vi "HandleClients.vi"(8 "error in (no error)":errorcluster, 11 "GuiderSetup in":refnum<class "GuiderSetup.lvclass">) -> (0 "error out":errorcluster, 3 "GuiderSetup out":refnum<class "GuiderSetup.lvclass">)   [LabVIEW 2018, in "GuiderSetup.lvclass"]
uses:
  GuiderSetup.lvclass
  C:/Users/devstaff/sparc4/s4gui/Versao ZeroMQ REQ-REP/SPARC4_GUI -v1.0.8 - reconhecimento do ACK do ACS/S4GUI/S4GUI.lvclass
  GuiderSetup.lvclass/GuiderSetup.ctl
  S4GUI/S4GUI.lvclass/S4GUI.ctl
  Instrument/Instrument.lvclass/Instrument.ctl
  Device/Optics/Optics.lvclass/Optics.ctl
  Device/Optics/Opt_Continuous/Opt_Continuous.lvclass
  C:/Users/devstaff/sparc4/s4gui/Versao ZeroMQ REQ-REP/SPARC4_GUI -v1.0.8 - reconhecimento do ACK do ACS/Device/Optics/Optics.lvclass
  Instrument/Instrument.lvclass
  Client_s4gui/Client_s4gui.lvclass
  PublisherGS/PublisherGS.lvclass
  AG/AG.lvclass
  S4GUI/S4GUI.lvclass
  Device/Optics/Optics.lvclass
  StateMachine/State Machine.lvclass
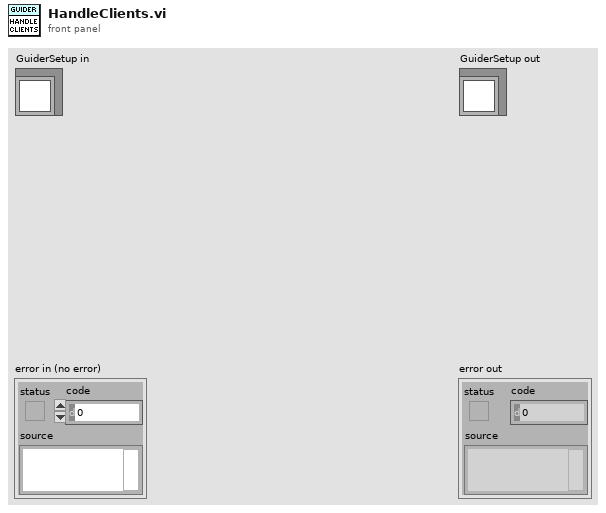
[diagram p1: front panel]
types:
  T1 = cluster{"FocusPhot":dbl, "FocusPolar":dbl, "FocusEffic":dbl, "FocusInstrum":dbl, "ICS":bool, "AG":bool, "broker":string, "timestamp":string, "FocusPos":dbl, "MirrorPos":dbl}
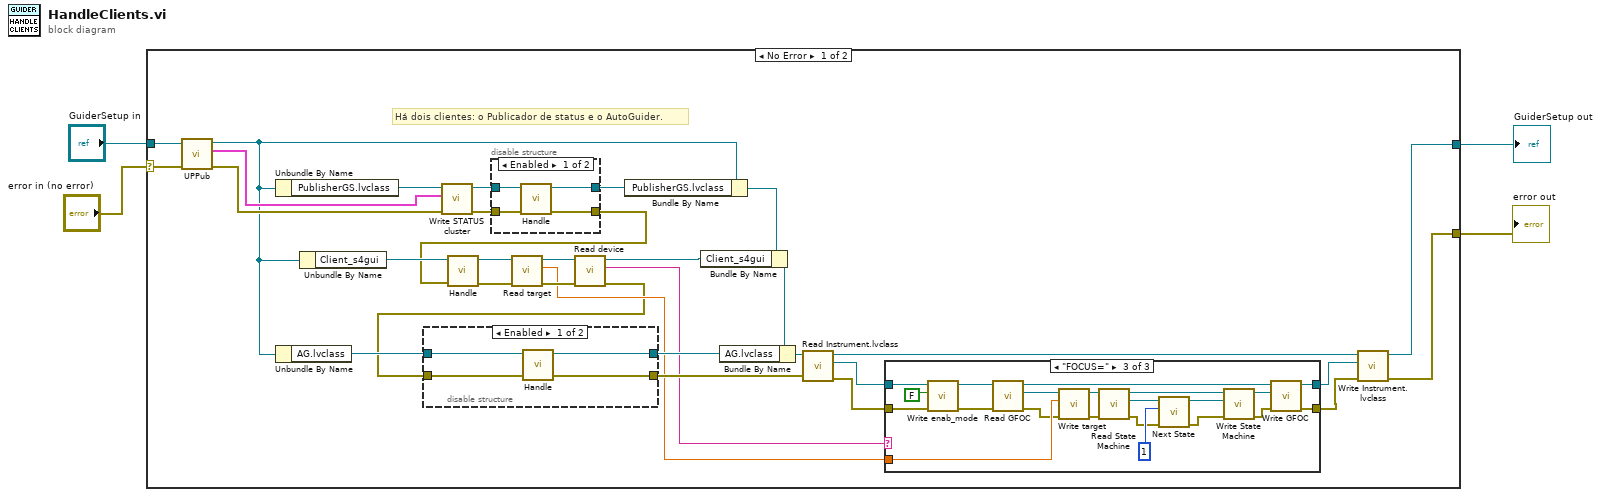
[diagram p0: block diagram]
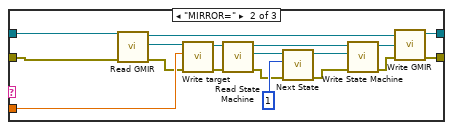
[diagram p3: hidden frame]
diagram:
  n1 = case shown="No Error" "error in (no error)" {
    selector: "error in (no error)" -> [w35 w90]
    tunnel: "GuiderSetup in" -> [w36 w91]
    tunnel: [w20 w91] -> w2
    tunnel: [w18 w90] -> w1
    frame No Error {
      # "Há dois clientes: o Publicador de status e o AutoGuider."
      n2 = call-dynamic "UPPub.vi"("error in (no error)"=w35, "GuiderSetup in"=w36) -> ("error out"=w31:errorcluster, "STATUS cluster"=w32:T1, "GuiderSetup out"=w26:refnum<class "GuiderSetup.lvclass">)  [unwired: 7 in]
      n3 = Unbundle By Name(w26) -> ("PublisherGS.lvclass"=w34:refnum<class "PublisherGS.lvclass">)
      n4 = Unbundle By Name(w26) -> ("AG.lvclass"=w28:refnum<class "AG.lvclass">)
      n5 = Unbundle By Name(w26) -> ("Client_s4gui"=w23:refnum<class "Client_s4gui.lvclass">)
      n6 = call-dynamic "Write STATUS cluster.vi"("error in (no error)"=w31, "STATUS cluster"=w32, "PublisherGS in"=w34) -> ("error out"=w30:errorcluster, "PublisherGS out"=w33:refnum<class "PublisherGS.lvclass">)  [unwired: 7 in]
      n7 = disable-structure shown="Enabled" {
        disable-tunnel: w33 -> [w81 w83]
        disable-tunnel: w30 -> [w80 w82]
        disable-tunnel: [w79 w83] -> w29
        disable-tunnel: [w78 w82] -> w6
        frame Enabled {
          n8 = call-dynamic "Handle.vi"("error in (no error)"=w80, "PublisherGS in"=w81) -> ("error out"=w78:errorcluster, "PublisherGS out"=w79:refnum<class "PublisherGS.lvclass">)  [unwired: 8 in]
        }
        frame Disabled {
        }
      }
      n9 = call-dynamic "Handle.vi"("error in (no error)"=w6, "Client_s4gui in"=w23) -> ("error out"=w14:errorcluster, "Client_s4gui out"=w17:refnum<class "Client_s4gui.lvclass">)  [unwired: 8 in]
      n10 = call-dynamic "Read target.vi"("error in (no error)"=w14, "Client_s4gui in"=w17) -> ("error out"=w13:errorcluster, "target"=w10:dbl, "Client_s4gui out"=w16:refnum<class "Client_s4gui.lvclass">)  [unwired: 7 in]
      n11 = call-dynamic "Read device.vi"("error in (no error)"=w13, "Client_s4gui in"=w16) -> ("error out"=w5:errorcluster, "device"=w11:string, "Client_s4gui out"=w15:refnum<class "Client_s4gui.lvclass">)  [unwired: 7 in]
      n12 = disable-structure shown="Enabled" {
        disable-tunnel: w28 -> [w87 w89]
        disable-tunnel: [w86 w89] -> w27
        disable-tunnel: w5 -> [w85 w88]
        disable-tunnel: [w84 w88] -> w19
        frame Enabled {
          n13 = call-dynamic "Handle.vi"("error in (no error)"=w85, "AG in"=w87) -> ("error out"=w84:errorcluster, "AG out"=w86:refnum<class "AG.lvclass">)  [unwired: 8 in]
        }
        frame Disabled {
        }
      }
      n14 = Bundle By Name(cluster=w26, "PublisherGS.lvclass"=w29) -> (w25:refnum<class "GuiderSetup.lvclass">)
      n15 = Bundle By Name(cluster=w25, "Client_s4gui"=w15) -> (w24:refnum<class "GuiderSetup.lvclass">)
      n16 = Bundle By Name(cluster=w24, "AG.lvclass"=w27) -> (w22:refnum<class "GuiderSetup.lvclass">)
      n17 = call "Read Instrument.lvclass.vi"("error in (no error)"=w19, "S4ACS_GUI in"=w22) -> ("error out"=w9:errorcluster, "Instrument.lvclass"=w12:refnum<class "Instrument.lvclass">, "S4ACS_GUI out"=w21:refnum<class "GuiderSetup.lvclass">)  [unwired: 7 in]
      n18 = case shown="\"FOCUS=\"" w11 {
        tunnel: w12 -> [w38 w54 w62]
        tunnel: w10 -> [_ w56 w77]
        tunnel: w9 -> [w37 w46 w59]
        tunnel: [w38 w40 w65] -> w8
        tunnel: [w37 w39 w64] -> w7
        frame Default {
        }
        frame "MIRROR=" {
          n19 = call "Read GMIR.vi"("error in (no error)"=w46, "Instrument in"=w54) -> ("error out"=w45:errorcluster, "Opt_Continuous.lvclass"=w52:refnum<class "Opt_Continuous.lvclass">, "Instrument out"=w53:refnum<class "Instrument.lvclass">)  [unwired: 7 in]
          n20 = call "Write target.vi"("error in (no error)"=w45, "target"=w56, "Optics in"=w52) -> ("error out"=w44:errorcluster, "Optics out"=w51:refnum<class "Opt_Continuous.lvclass">)  [unwired: 7 in]
          n21 = call-dynamic "Read State Machine.vi"("error in (no error)"=w44, "Device in"=w51) -> ("error out"=w43:errorcluster, "State Machine.lvclass"=w49:refnum<class "State Machine.lvclass">, "Device out"=w50:refnum<class "Opt_Continuous.lvclass">)  [unwired: 7 in]
          n22 = call "Next State.vi"("error in (no error)"=w43, "New_State"=1, "State Machine in"=w49) -> ("error out"=w42:errorcluster, "State Machine out"=w48:refnum<class "State Machine.lvclass">)  [unwired: 7 in]
          n23 = call-dynamic "Write State Machine.vi"("error in (no error)"=w42, "State Machine.lvclass"=w48, "Device in"=w50) -> ("error out"=w41:errorcluster, "Device out"=w47:refnum<class "Opt_Continuous.lvclass">)  [unwired: 7 in]
          n24 = call "Write GMIR.vi"("error in (no error)"=w41, "Opt_Continuous.lvclass"=w47, "Instrument in"=w53) -> ("error out"=w39:errorcluster, "Instrument out"=w40:refnum<class "Instrument.lvclass">)  [unwired: 7 in]
        }
        frame "FOCUS=" {
          n25 = call-dynamic "Write enab_mode.vi"("error in (no error)"=w59, "enab_mode"=FALSE, "Instrument in"=w62) -> ("error out"=w60:errorcluster, "Instrument out"=w61:refnum<class "Instrument.lvclass">)  [unwired: 7 in]
          n26 = call "Read GFOC.vi"("error in (no error)"=w60, "Instrument in"=w61) -> ("error out"=w58:errorcluster, "Opt_Continuous.lvclass"=w57:refnum<class "Opt_Continuous.lvclass">, "Instrument out"=w75:refnum<class "Instrument.lvclass">)  [unwired: 7 in]
          n27 = call "Write target.vi"("error in (no error)"=w58, "target"=w77, "Optics in"=w57) -> ("error out"=w69:errorcluster, "Optics out"=w74:refnum<class "Opt_Continuous.lvclass">)  [unwired: 7 in]
          n28 = call-dynamic "Read State Machine.vi"("error in (no error)"=w69, "Device in"=w74) -> ("error out"=w68:errorcluster, "State Machine.lvclass"=w72:refnum<class "State Machine.lvclass">, "Device out"=w73:refnum<class "Opt_Continuous.lvclass">)  [unwired: 7 in]
          n29 = call "Next State.vi"("error in (no error)"=w68, "New_State"=1, "State Machine in"=w72) -> ("error out"=w67:errorcluster, "State Machine out"=w71:refnum<class "State Machine.lvclass">)  [unwired: 7 in]
          n30 = call-dynamic "Write State Machine.vi"("error in (no error)"=w67, "State Machine.lvclass"=w71, "Device in"=w73) -> ("error out"=w66:errorcluster, "Device out"=w70:refnum<class "Opt_Continuous.lvclass">)  [unwired: 7 in]
          n31 = call "Write GFOC.vi"("error in (no error)"=w66, "Opt_Continuous.lvclass"=w70, "Instrument in"=w75) -> ("error out"=w64:errorcluster, "Instrument out"=w65:refnum<class "Instrument.lvclass">)  [unwired: 7 in]
        }
      }
      n32 = call "Write Instrument.lvclass.vi"("error in (no error)"=w7, "Instrument.lvclass"=w8, "S4ACS_GUI in"=w21) -> ("error out"=w18:errorcluster, "S4ACS_GUI out"=w20:refnum<class "GuiderSetup.lvclass">)  [unwired: 7 in]
    }
    frame Error {
    }
  }
  "error out" <- w1
  "GuiderSetup out" <- w2
